vi "Write Char Register.vi"(7 "PDU Address Char 8-bit":T1 items=["Wink"=0, "Control mode"=36, "Alarm mode"=3107, "Alarm setpoint"=3109, "Reset alarm enable"=3113, "Counter setpoint mode"=3333, "Reset counter enable"=3337, "Modbus slave address"=4010], 8 "error in":errorcluster, 10 "Unsigned Char":string, 11 "MB_TCP session in":refnum<class "MB_Master_TCP.lvclass">) -> (0 "error out":errorcluster, 3 "MB session out":refnum<class "MB_Master_TCP.lvclass">)   [LabVIEW 2024, in "Bronkhorst Flexi-Flow ModbusTCP API.lvlib"]
uses:
  Bronkhorst Flexi-Flow ModbusTCP API.lvlib
  <vilib>/Plasmionique/MB Master/MB_Master_TCP/MB_Master_TCP.lvclass
  C:/Program Files/National Instruments/LabVIEW 2025/vi.lib/Plasmionique/MB Master/MB_Master/MB_Master.lvclass
  PDU Address Char 8-bit Params--ring.ctl
  <vilib>/Plasmionique/MB Master/MB Master.lvlib
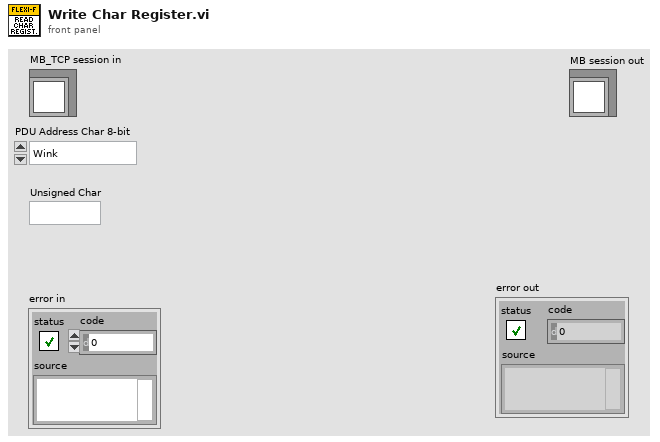
[diagram p1: front panel]
types:
  T1 = typedef "Bronkhorst Flexi-Flow ModbusTCP API.lvlib/PDU Address Char 8-bit Params--ring.ctl" = u16
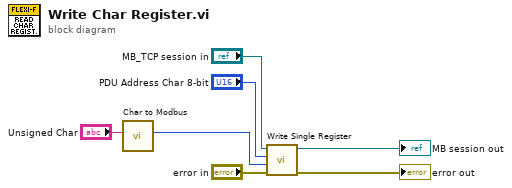
[diagram p0: block diagram]
diagram:
  n1 = call "Char to Modbus.vi"("Unsigned Char"="Unsigned Char") -> ("Char Register Out"=w1:u16)  [unwired: 10 in]
  n2 = call <vilib>:"Write Single Register.vi"("error in (no error)"="error in", "value"=w1, "address"="PDU Address Char 8-bit", "MB session in"="MB_TCP session in") -> ("error out"=→"error out":errorcluster, "MB session out"=→"MB session out":refnum<class "MB_Master_TCP.lvclass">)  [unwired: 6 in]
